vi "Set Uim ICFG wrapper.vi"(7 "bAckEna":i32, 8 "error in (no error)":errorcluster caption="错误输入（无错误）", 9 "UIM_ICFG_INFO_OBJ In":T1, 10 "dwCanNodeId":u32, 11 "dwDevIndex":u32) -> (0 "error out":errorcluster caption="错误输出", 1 "UIM_ICFG_INFO_OBJ Out":T1, 3 "function return":u32)   [LabVIEW 2016, in "UISimCanFunc_wrapper.lvlib"]
doc: "_declspec (dllexport) DWORD SetUimICFG_wrapper(DWORD dwDevIndex, DWORD dwCanNodeId,\n P_DUMMY_UIM_ICFG_INFO_OBJ pDummyICFGInfoIn, BOOL bAckEna, P_DUMMY_UIM_ICFG_INFO_OBJ pDummyICFGInfoOut);"
uses:
  <userlib>/UISimCanFunc_wrapper/UISimCanFunc_wrapper.lvlib
  <userlib>/UISimCanFunc_wrapper/ctl/UIM_ICFG_INFO_OBJ.ctl
  <userlib>/UISimCanFunc_wrapper/UISimCanFunc_wrapper.dll
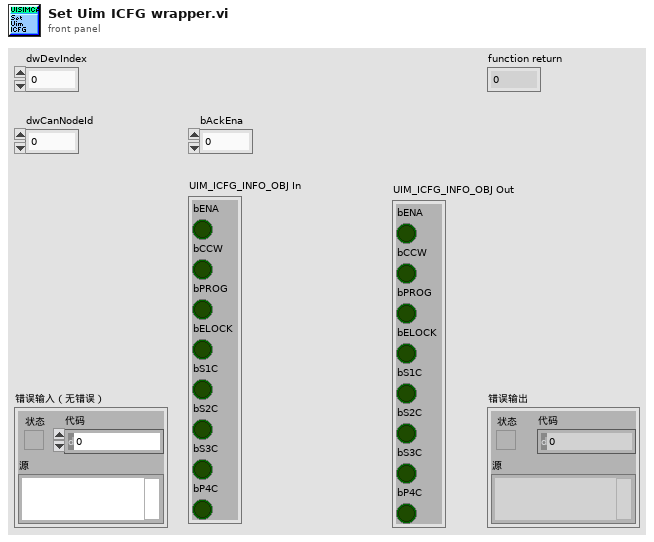
[diagram p1: front panel]
types:
  T1 = typedef "UISimCanFunc_wrapper.lvlib/UIM_ICFG_INFO_OBJ.ctl" = cluster{"bENA":bool, "bCCW":bool, "bPROG":bool, "bELOCK":bool, "bS1C":bool, "bS2C":bool, "bS3C":bool, "bP4C":bool}
  T2 = cluster{"bENA":i32, "bCCW":i32, "bPROG":i32, "bELOCK":i32, "bS1C":i32, "bS2C":i32, "bS3C":i32, "bP4C":i32}
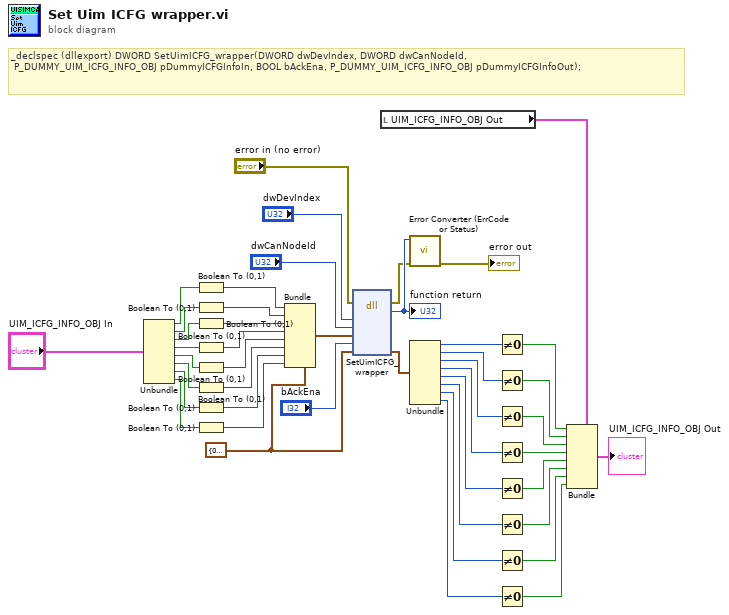
[diagram p0: block diagram]
diagram:
  w17 = T2 {"bENA"=0, "bCCW"=0, "bPROG"=0, "bELOCK"=0, "bS1C"=0, "bS2C"=0, "bS3C"=0, "bP4C"=0} ("pDummyICFGInfoOut")
  # "_declspec (dllexport) DWORD SetUimICFG_wrapper(DWORD dwDevIndex, DWORD dwCanNodeId,\n\tP_DUMMY_UIM_ICFG_INFO_OBJ pDummyICFGInfoIn, BOOL bAckEna, P_DUMMY_UIM_ICFG_INFO_OBJ pDummyICFGInfoOut);"
  n1 = Unbundle("UIM_ICFG_INFO_OBJ In") -> ("bENA"=w37:bool, "bCCW"=w36:bool, "bPROG"=w35:bool, "bELOCK"=w34:bool, "bS1C"=w16:bool, "bS2C"=w15:bool, "bS3C"=w14:bool, "bP4C"=w13:bool)
  n2 = Boolean To (0,1)(Boolean=w37) -> (0, 1=w33:i16)
  n3 = Boolean To (0,1)(Boolean=w36) -> (0, 1=w32:i16)
  n4 = Boolean To (0,1)(Boolean=w35) -> (0, 1=w31:i16)
  n5 = Boolean To (0,1)(Boolean=w34) -> (0, 1=w30:i16)
  n6 = Boolean To (0,1)(Boolean=w16) -> (0, 1=w12:i16)
  n7 = Boolean To (0,1)(Boolean=w15) -> (0, 1=w11:i16)
  n8 = Boolean To (0,1)(Boolean=w14) -> (0, 1=w10:i16)
  n9 = Boolean To (0,1)(Boolean=w13) -> (0, 1=w9:i16)
  n10 = Bundle(cluster=w17, "bENA"=w33, "bCCW"=w32, "bPROG"=w31, "bELOCK"=w30, "bS1C"=w12, "bS2C"=w11, "bS3C"=w10, "bP4C"=w9) -> (w29:T2)
  n11 = dll-call lib="C:/Program Files (x86)/National Instruments/LabVIEW 2016/user.lib/UISimCanFunc_wrapper/UISimCanFunc_wrapper.*" fn="SetUimICFG_wrapper"(error in="error in (no error)", "dwDevIndex"="dwDevIndex", "dwCanNodeId"="dwCanNodeId", "pDummyICFGInfoIn"=w29, "bAckEna"="bAckEna", "pDummyICFGInfoOut"=w17) -> (error out=w40:errorcluster, w45:u32, "pDummyICFGInfoOut"=w19:T2)  [unwired: 6 in, 1 out]
  "function return" <- w45
  n12 = local read "UIM_ICFG_INFO_OBJ Out"() -> (w18:T1)
  n13 = call <userlib>:"Error Converter (ErrCode or Status).vi"("error in (no error)"=w40, "error code"=w45) -> ("error out"=→"error out":errorcluster)  [unwired: 9 in]
  n14 = Unbundle(w19) -> ("bENA"=w27:i32, "bCCW"=w26:i32, "bPROG"=w25:i32, "bELOCK"=w24:i32, "bS1C"=w8:i32, "bS2C"=w7:i32, "bS3C"=w6:i32, "bP4C"=w5:i32)
  n15 = Not Equal To 0?(x=w27) -> (x != 0?=w23:bool)
  n16 = Not Equal To 0?(x=w26) -> (x != 0?=w22:bool)
  n17 = Not Equal To 0?(x=w25) -> (x != 0?=w21:bool)
  n18 = Not Equal To 0?(x=w24) -> (x != 0?=w20:bool)
  n19 = Not Equal To 0?(x=w8) -> (x != 0?=w4:bool)
  n20 = Not Equal To 0?(x=w7) -> (x != 0?=w3:bool)
  n21 = Not Equal To 0?(x=w6) -> (x != 0?=w2:bool)
  n22 = Not Equal To 0?(x=w5) -> (x != 0?=w1:bool)
  n23 = Bundle(cluster=w18, "bENA"=w23, "bCCW"=w22, "bPROG"=w21, "bELOCK"=w20, "bS1C"=w4, "bS2C"=w3, "bS3C"=w2, "bP4C"=w1) -> (→"UIM_ICFG_INFO_OBJ Out":T1)
